vi "load Example Script.vi"(8 "error in (no error)":errorcluster) -> (0 "error out":errorcluster)   [LabVIEW 2014, in "exampleWrapper.lvlib"]
doc: "void loadExampleScript(void)"
uses:
  exampleWrapper.lvlib
  <userlib>/exampleWrapper/exampleWrapper.dll
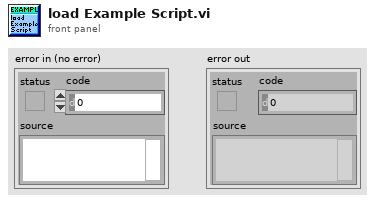
[diagram p1: front panel]
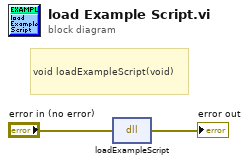
[diagram p0: block diagram]
diagram:
  # "void loadExampleScript(void)"
  n1 = dll-call lib="C:/Program Files/National Instruments/LabVIEW 2018/user.lib/exampleWrapper/exampleWrapper.*" fn="loadExampleScript"(error in="error in (no error)") -> (error out=→"error out":errorcluster)  [unwired: 3 in, 1 out]
